vi "Set message.vi"(10 "WampMessage JSON":refnum<class "WampMessage JSON.lvclass">, 11 "ErrorHandler JSON in":refnum<class "ErrorHandler JSON.lvclass">) -> (3 "ErrorHandler JSON out":refnum<class "ErrorHandler JSON.lvclass">)   [LabVIEW 2020, in "wamplv.lvlib" / "ErrorHandler JSON.lvclass"]
uses:
  ErrorHandler JSON.lvclass
  ErrorHandler JSON.lvclass/ErrorHandler JSON.ctl
  SerialisedMessages/JSONMessage/WampMessage JSON.lvclass
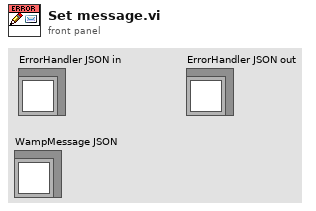
[diagram p1: front panel]
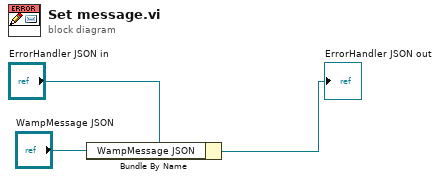
[diagram p0: block diagram]
diagram:
  n1 = Bundle By Name(cluster="ErrorHandler JSON in", "WampMessage JSON"="WampMessage JSON") -> (→"ErrorHandler JSON out":refnum<class "ErrorHandler JSON.lvclass">)
